vi "JoystickControls.vi"() -> (3 "output cluster":T1)   [LabVIEW 2015]
uses:
  Controls.ctl
  References/Refnums.vi
  <vilib>/Rock Robotics/WPI/Utilities/WPI_GetSetVariantRefNum.vi
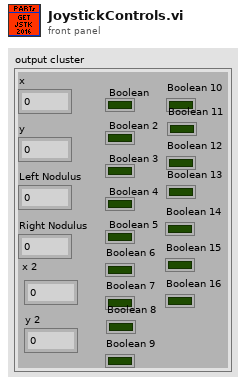
[diagram p1: front panel]
types:
  T1 = typedef "Controls.ctl" = cluster{"x":dbl, "y":dbl, "Left Nodulus":dbl, "Right Nodulus":dbl, "Boolean":bool, "Boolean 2":bool, "Boolean 3":bool, "Boolean 4":bool, "Boolean 5":bool, "Boolean 6":bool, "Boolean 7":bool, "Boolean 8":bool, "Boolean 9":bool, "Boolean 10":bool, "Boolean 11":bool, "Boolean 12":bool, "Boolean 13":bool, "Boolean 14":bool, "Boolean 15":bool, "x 2":dbl, "y 2":dbl, "Boolean 16":bool}
  T2 = typedef "WPI_JoystickDevRef.ctl" = cluster{"Device":T3}
  T3 = typedef "WPI_JoystickDeviceEnum.ctl" = enum16{"USB 0", "USB 1", "USB 2", "USB 3", "USB 4", "USB 5"}
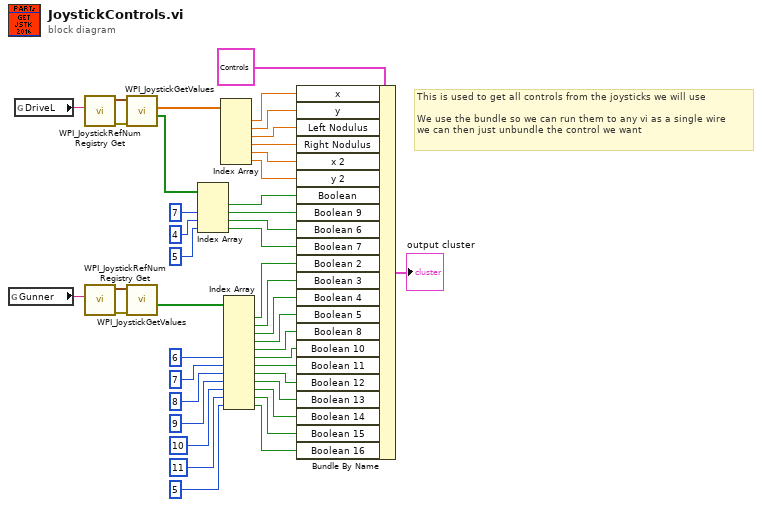
[diagram p0: block diagram]
diagram:
  # "This is used to get all controls from the joysticks we will use\n\nWe use the bundle so we can run them to any vi as a single wire\nwe can then just unbundle the control we want"
  n1 = global read "Refnums.vi" "Gunner"() -> (w42:string)
  n2 = global read "Refnums.vi" "DriveL"() -> (w37:string)
  n3 = call <vilib>:"WPI_JoystickRefNum Registry Get.vi"("refnum name"=w37) -> ("error out"=w35:errorcluster, "JoystickDevRef"=w36:T2)  [unwired: 9 in]
  n4 = call <vilib>:"WPI_JoystickRefNum Registry Get.vi"("refnum name"=w42) -> ("error out"=w40:errorcluster, "JoystickDevRef"=w41:T2)  [unwired: 9 in]
  n5 = call <vilib>:"WPI_JoystickGetValues.vi"("error in (no error)"=w35, "JoystickDevRef"=w36) -> ("Buttons"=w33:bool[], "Axes"=w34:dbl[])  [unwired: 5 in, 3 out]
  n6 = call <vilib>:"WPI_JoystickGetValues.vi"("error in (no error)"=w40, "JoystickDevRef"=w41) -> ("Buttons"=w43:bool[])  [unwired: 5 in, 4 out]
  n7 = Index Array(array=w33, index #2=7 ("index"), index #3=4 ("index"), index #4=5 ("index")) -> (element #1=w32:bool, element #2=w30:bool, element #3=w27:bool, element #4=w26:bool)  [unwired: 1 in]
  n8 = Index Array(array=w34) -> (element #1=w3:dbl, element #2=w4:dbl, element #3=w5:dbl, element #4=w6:dbl, element #5=w7:dbl, element #6=w8:dbl)  [unwired: 6 in]
  n9 = Index Array(array=w43, index #6=6 ("index"), index #7=7 ("index"), index #8=8 ("index"), index #9=9 ("index"), index #10=10 ("index"), index #11=11 ("index"), index #12=5 ("index")) -> (element #1=w25:bool, element #2=w24:bool, element #3=w23:bool, element #4=w22:bool, element #5=w21:bool, element #6=w19:bool, element #7=w17:bool, element #8=w15:bool, element #9=w13:bool, element #10=w11:bool, element #11=w9:bool, element #12=w1:bool)  [unwired: 5 in]
  n10 = Bundle By Name(cluster=T1 {"x"=0.0, "y"=0.0, "Left Nodulus"=0.0, "Right Nodulus"=0.0, "Boolean"=FALSE, "Boolean 2"=FALSE, "Boolean 3"=FALSE, "Boolean 4"=FALSE, "Boolean 5"=FALSE, "Boolean 6"=FALSE, "Boolean 7"=FALSE, "Boolean 8"=FALSE, "Boolean 9"=FALSE, "Boolean 10"=FALSE, "Boolean 11"=FALSE, "Boolean 12"=FALSE, "Boolean 13"=FALSE, "Boolean 14"=FALSE, "Boolean 15"=FALSE, "x 2"=0.0, "y 2"=0.0, "Boolean 16"=FALSE} ("input cluster"), "x"=w3, "y"=w4, "Left Nodulus"=w5, "Right Nodulus"=w6, "x 2"=w7, "y 2"=w8, "Boolean"=w32, "Boolean 9"=w30, "Boolean 6"=w27, "Boolean 7"=w26, "Boolean 2"=w25, "Boolean 3"=w24, "Boolean 4"=w23, "Boolean 5"=w22, "Boolean 8"=w21, "Boolean 10"=w19, "Boolean 11"=w17, "Boolean 12"=w15, "Boolean 13"=w13, "Boolean 14"=w11, "Boolean 15"=w9, "Boolean 16"=w1) -> (→"output cluster":T1)
